vi "Read LeafData.vi"(8 "error in (no error)":errorcluster caption="错误输入（无错误）", 11 "PanelRootNode 输入":refnum<class "PanelRootNode.lvclass"> caption="DNL_LabVIEW Object in") -> (0 "error out":errorcluster caption="错误输出", 2 "数组":variant[](array[variant]), 3 "PanelRootNode 输出":refnum<class "PanelRootNode.lvclass"> caption="DNL_LabVIEW Object out")   [LabVIEW 2013, in "PanelRootNode.lvclass"]
uses:
  PanelRootNode.lvclass
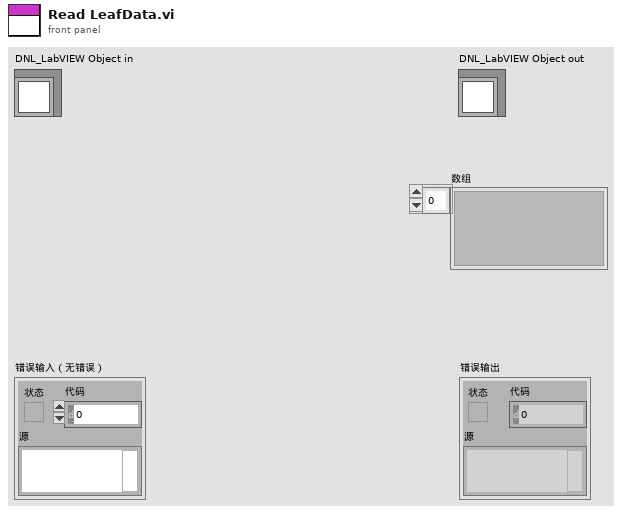
[diagram p1: front panel]
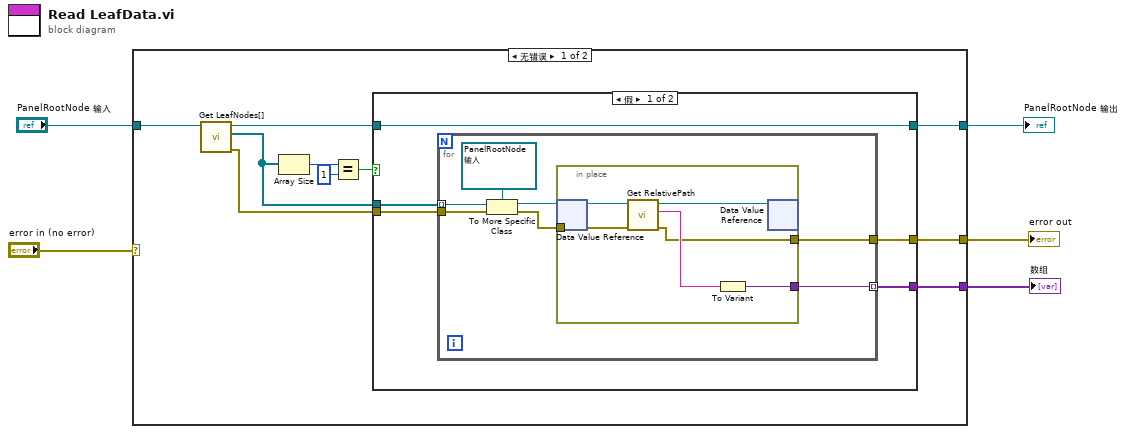
[diagram p0: block diagram]
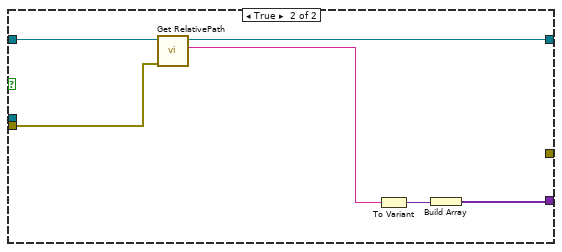
[diagram p2: hidden frame]
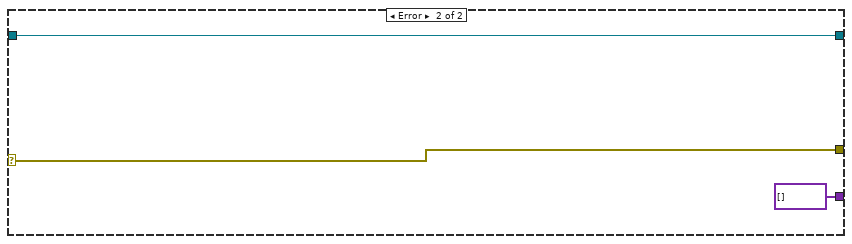
[diagram p3: hidden frame]
diagram:
  n1 = case shown="无错误" "error in (no error)" {
    selector: "error in (no error)" -> [_ w42]
    tunnel: [w6 w42] -> w4
    tunnel: [w12 w41] -> w2
    tunnel: "PanelRootNode 输入" -> [w9 w41]
    tunnel: [w8 variant[] []] -> w1
    frame No Error {
      n2 = call "Get LeafNodes[].vi"("PanelRootNode 输入"=w9) -> ("error out"=w7:errorcluster, "LeafNodes[]"=w10:refnum<data-value>[], "PanelRootNode 输出"=w13:refnum<class "PanelRootNode.lvclass">)  [unwired: 8 in]
      n3 = Array Size(array=w10) -> (size(s)=w15:i32)
      n4 = Equal?(x=w15, y=1) -> (x = y?=w11:bool)
      n5 = case shown="假" w11 {
        tunnel: w13 -> [w20 w39]
        tunnel: [w20 w38] -> w12
        tunnel: w10 -> [w19 _]
        tunnel: [w18 w35] -> w8
        tunnel: w7 -> [w17 w34]
        tunnel: [w16 _] -> w6
        frame False {
          n6 = for {
            tunnel: w19 -> [w27] mode=indexing
            tunnel: [w24] -> w18 mode=indexing
            tunnel: w17 -> [w23]
            tunnel: [w21] -> w16
            n7 = To More Specific Class(target class=refnum<data-value> refnum ("数据值引用"), reference=w27, error in=w23) -> (specific class reference=w25:refnum<data-value>, error out=w22:errorcluster)
            n8 = in-place {
              in-place-border: [w30] -> w24
              in-place-border: w22 -> [w29]
              in-place-border: [w28] -> w21
              n9 = in-place-dvr #1(w25) -> (w33:refnum<class "PanelRootNode.lvclass">)  [unwired: 1 out]
              n10 = call "Get RelativePath.vi"("error in (no error)"=w29, "PanelRootNode 输入"=w33) -> ("error out"=w28:errorcluster, "RelativePath"=w31:string, "PanelRootNode 输出"=w32:refnum<class "PanelRootNode.lvclass">)  [unwired: 7 in]
              n11 = To Variant(anything=w31) -> (Variant=w30:variant)
              n12 = in-place-dvr #1(w32) -> ()  [unwired: 2 out]
            }
          }
        }
        frame True {
          n13 = call "Get RelativePath.vi"("error in (no error)"=w34, "PanelRootNode 输入"=w39) -> ("RelativePath"=w37:string, "PanelRootNode 输出"=w38:refnum<class "PanelRootNode.lvclass">)  [unwired: 7 in, 1 out]
          n14 = To Variant(anything=w37) -> (Variant=w36:variant)
          n15 = Build Array(w36) -> (w35:variant[])
        }
      }
    }
    frame Error {
    }
  }
  "error out" <- w4
  "PanelRootNode 输出" <- w2
  "数组" <- w1
